vi "TLB Native Dynamic Events ver 0.10.vi"() -> ()   [LabVIEW 2018]
uses:
  Labview Training Phase 2/Enum Controls/States for Action Engine.ctl
  TLB Type Definitions/State Type Definitions.ctl
  TLB Type Definitions/Intruction Type Definitions.ctl
  TLB Type Definitions/Encoder cluster.ctl
  Experimental VI's/Archived VI's/MOTOR CONTROL NO PID Type Def.ctl
  Underlying VI's/I2C Master VI/I2C MASTER Type Def.ctl
  TLB Type Definitions/PING CLUSTER.ctl
  <vilib>/Studica/Studica Toolkit/NavX/NavX.lvlib
  <vilib>/Studica/Studica Toolkit/Background/DIO Channel.ctl
panel:
  out "Object detected?":bool
  out "TASK ENABLE":bool
  out "Rising Edge":bool
  in  "Green LED":bool
  out "Timestamp":u32
  out "NavX Output":T1
  in  "Zero Yaw":bool
  out "Task Selection":u8
  out "Object detected?":bool
  in  "Arduino Mode":T2=enum."Mode 0"
  out "Arduino Data":T3
  out "I2C Error":errorcluster
  out "Speed & distance":T4
  out "State Logic":T5=enum."Startup"
  out "elements":T6[](array[typedef])
  in  "STOP TASK":bool
  in  "OK Button":bool
  in  "STOP":bool
  out "error out":errorcluster
  out "Action Queue Items":i32
  out "State Logic Queue Items":i32
  out "Action Queues items":string[](array[string])=["Hardware reset", "Software reset", ""]
  out "Action State":string
  # "TLB FRAMEWORK STATUS"
  # "System Health Status Update"
  # "Test Programme written by Calvin Loke    Dated: 28 Aug 2019\nTest Programme revised by Dr Alex See   Dated 30 Aug 2019\n\nProgramme version:   TLB Native Dynamic Events ver 0.04b.vi"
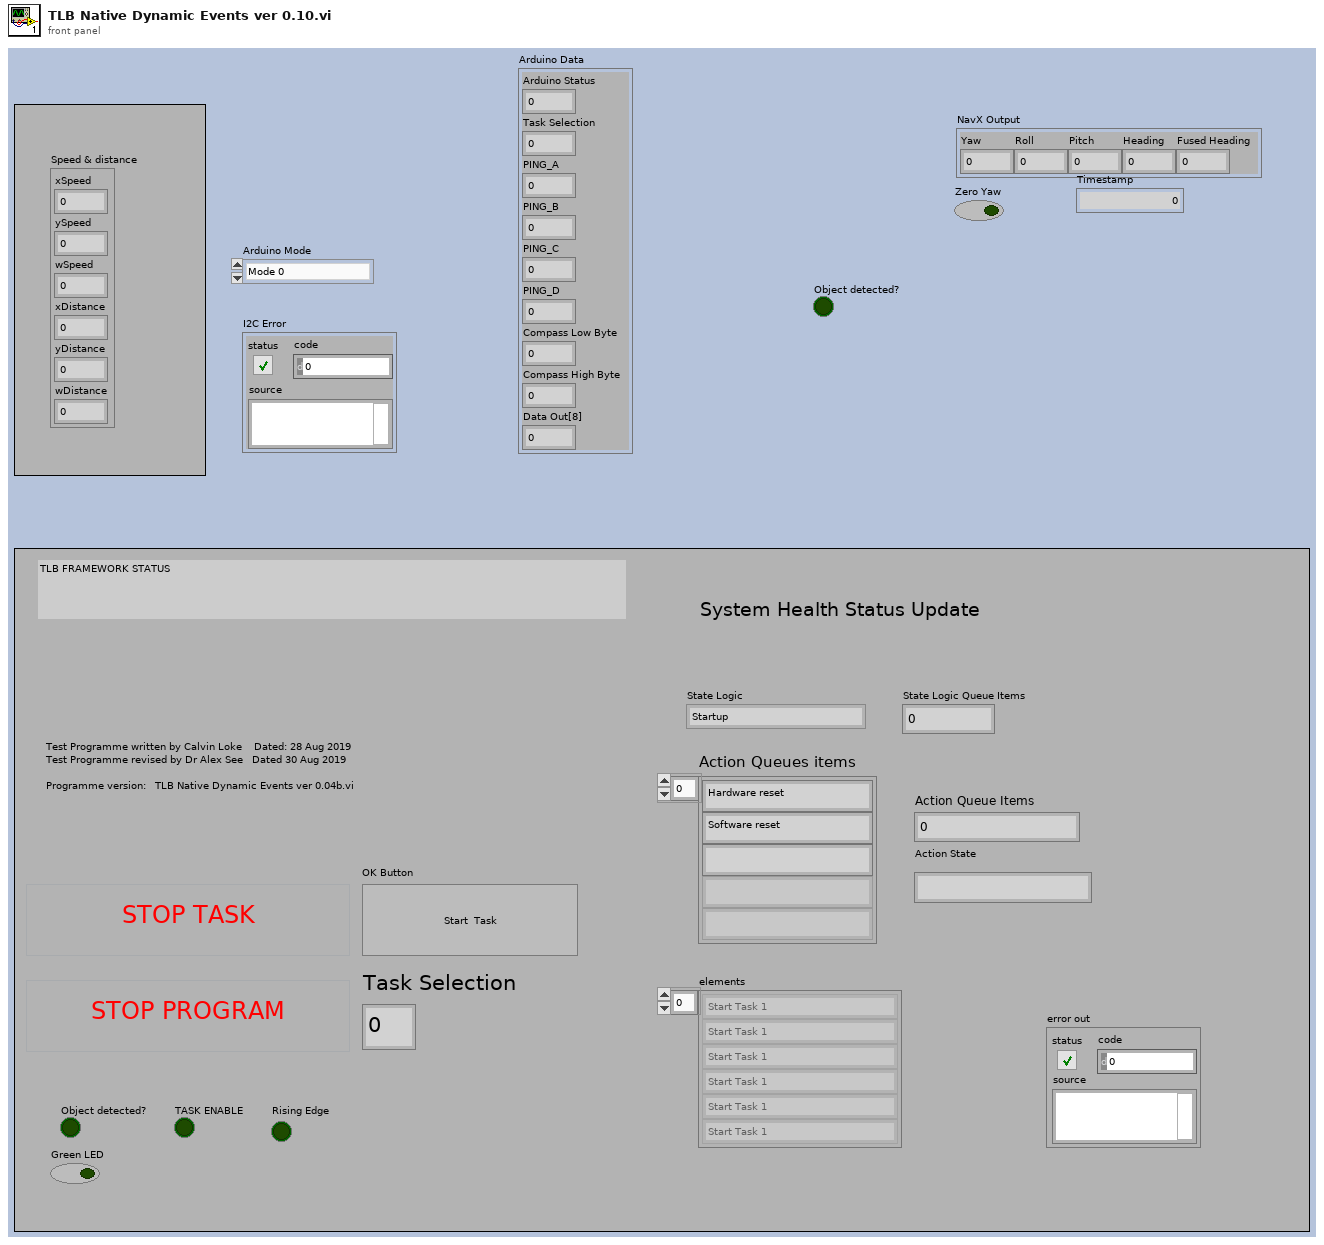
[diagram p1: front panel]
types:
  T1 = cluster{"Yaw":dbl, "Roll":dbl, "Pitch":dbl, "Heading":dbl, "Fused Heading":dbl}
  T2 = typedef "I2C MASTER Type Def.ctl" = enum16{"Last State", "Mode 0", "Mode 1", "Mode 2", "Mode 3", "Mode 4", "Mode 5", "Mode 6", "Mode 7", "Mode 8", "Mode 9", "Mode 10"}
  T3 = cluster{"Arduino Status":u8, "Task Selection":u8, "PING_A":u8, "PING_B":u8, "PING_C":u8, "PING_D":u8, "Compass Low Byte":u8, "Compass High Byte":u8, "Data Out[8]":u8}
  T4 = cluster{"xSpeed":dbl, "ySpeed":dbl, "wSpeed":dbl, "xDistance":dbl, "yDistance":dbl, "wDistance":dbl}
  T5 = typedef "State Type Definitions.ctl" = enum16{"None", "Startup", "Move to Angle", "True Stop", "Idle", "Shutdown", "Task 1A", "Task 1B", "Task 2:Raise Arm", "Task 2:Sensor Mode", "Task 2:Reverse Mode", "Task 3", "Task 4_A", "Task 4_B", "Task 4_C", "Task 4_D", "Task 5A", "Task 5B", "Task 5C", "Task 5D", "Task 5E: POSITION ARM", "Task 5F: ARM GRAB HEIGHT", "Task 5G: CLOSE CLAW", "Task 5H: RAISE ARM", "Task 6_A", "Task 6_B", "Task 7", "Task 8A: RAISE ARM", "Task 8B: MOVE TO BOX", "Task 8C: CAM BURST", "Task 8D: PROCESS IMAGE", "Task 8E: ROBOT ADJUST", "Task 8F: CAM BURST 2", "Task 8G: PROCESS IMAGE 2", "Task 8H: ARM ADJUST", "Task 8I: ARM GRAB HEIGHT", "Task 8J: CLOSE CLAW", "Task 8K: RAISE MY SWORD", "Task 9A: Raise Arm", "Task 9B: Rotate to Angle", "Task 9C: Detect Box", "Task 9D: MOVE FORWARD", "Task 9E: MOVE LEFT", "Task 9F: SCAN IMAGE", "Task 9G: PROCESS COLOUR", "Task 9H: MOVE RIGHT", "Task 9I: SCAN IMAGE", "Task 9J: PROCESS COLOUR", "Task 9K: ROTATE 90 CW", "Task 9L: MOVE FORWARD", "Task 9M: MOVE RIGHT", "Task 9N: SCAN IMAGE", "Task 9O: PROCESS COLOUR", "Task 9P: MOVE RIGHT", "Task 9Q: SCAN IMAGE", "Task 9R: PROCESS COLOUR"}
  T6 = typedef "Intruction Type Definitions.ctl" = enum16{"None", "Start Task 1", "Start Task 2", "Start Task 3", "Start Task 4", "Start Task 5", "Start Task 6", "Start Task 7", "Start Task 8 - BALL", "Start Task 8 - Gel", "Start Task 8 - Pipe", "Start Task 8 - Soap", "Start Task 9", "Start Task A", "Start Task B", "Exit"}
  T7 = typedef "States for Action Engine.ctl" = enum16{"Initialize", "Write", "Read"}
  T8 = typedef "DIO Channel.ctl" = enum16{"Not Connected", "A/DIO1", "A/DIO2", "A/DIO3", "A/DIO4", "A/DIO5", "A/DIO6", "A/DIO7", "A/DIO13", "B/DIO1", "B/DIO2", "B/DIO3", "B/DIO4", "B/DIO5", "B/DIO6", "B/DIO7", "B/DIO13", "C/DIO0", "C/DIO1", "C/DIO2", "C/DIO3", "C/DIO4", "C/DIO5", "C/DIO6", "C/DIO7"}
  T9 = typedef "PING CLUSTER.ctl" = cluster{"PING_A":u8, "PING_B":u8, "PING_C":u8, "PING_D":u8}
  T10 = typedef "Encoder cluster.ctl" = cluster{"xDistance":dbl, "yDistance":dbl, "wDistance":dbl}
  T11 = typedef "State Type Definitions.ctl" = enum16{"None", "Startup", "Move to Angle", "True Stop", "Idle", "Shutdown", "Task 1", "Task 2:Raise Arm", "Task 2:Sensor Mode", "Task 2:Reverse Mode", "Task 3", "Task 4_A", "Task 4_B", "Task 4_C", "Task 4_D", "Task 5A: ARM CAM HEIGHT", "Task 5B: MOVE TO BOX", "Task 5C: CAM BURST", "Task 5D: PROCESS IMAGE", "Task 5E: POSITION ARM", "Task 5F: ARM GRAB HEIGHT", "Task 5G: CLOSE CLAW", "Task 5H: RAISE ARM", "Task 6_A", "Task 6_B", "Task 7", "Task 8A: RAISE ARM", "Task 8B: MOVE TO BOX", "Task 8C: CAM BURST", "Task 8D: PROCESS IMAGE", "Task 8E: ROBOT ADJUST", "Task 8F: CAM BURST 2", "Task 8G: PROCESS IMAGE 2", "Task 8H: ARM ADJUST", "Task 8I: ARM GRAB HEIGHT", "Task 8J: CLOSE CLAW", "Task 8K: RAISE MY SWORD", "Task 9A: Raise Arm", "Task 9B: Rotate to Angle", "Task 9C: Detect Box", "Task 9D: MOVE FORWARD", "Task 9E: MOVE LEFT", "Task 9F: SCAN IMAGE", "Task 9G: PROCESS COLOUR", "Task 9H: MOVE RIGHT", "Task 9I: SCAN IMAGE", "Task 9J: PROCESS COLOUR", "Task 9K: ROTATE 90 CW", "Task 9L: MOVE FORWARD", "Task 9M: MOVE RIGHT", "Task 9N: SCAN IMAGE", "Task 9O: PROCESS COLOUR", "Task 9P: MOVE RIGHT", "Task 9Q: SCAN IMAGE", "Task 9R: PROCESS COLOUR"}
  T12 = typedef "State Type Definitions.ctl" = enum16{"None", "Startup", "Move to Angle", "True Stop", "Idle", "Shutdown", "Task 1", "Task 2", "Task 3", "Task 4_A", "Task 4_B", "Task 4_C", "Task 5", "Task 6", "Task 7", "Task 8", "Task 9", "Task A", "Task B"}
  T13 = typedef "MOTOR CONTROL NO PID Type Def.ctl" = enum16{"Init", "Front Back", "Left Right", "Rotate", "Stop", "Latch"}
  T14 = cluster{"DIO Channel":T8, "FPGA VI Reference Out":refnum<k20>}
  T15 = typedef "I2C Channel.ctl" = enum16{"Not Connected", "A", "B"}
  T16 = cluster{"I2C Ref Out":cluster{"I2C Channel":T15, "FPGA VI Reference Out":refnum<k20>}, "Connected":bool, "Slave Address (7-bit)":u8, "Registry":u8[]}
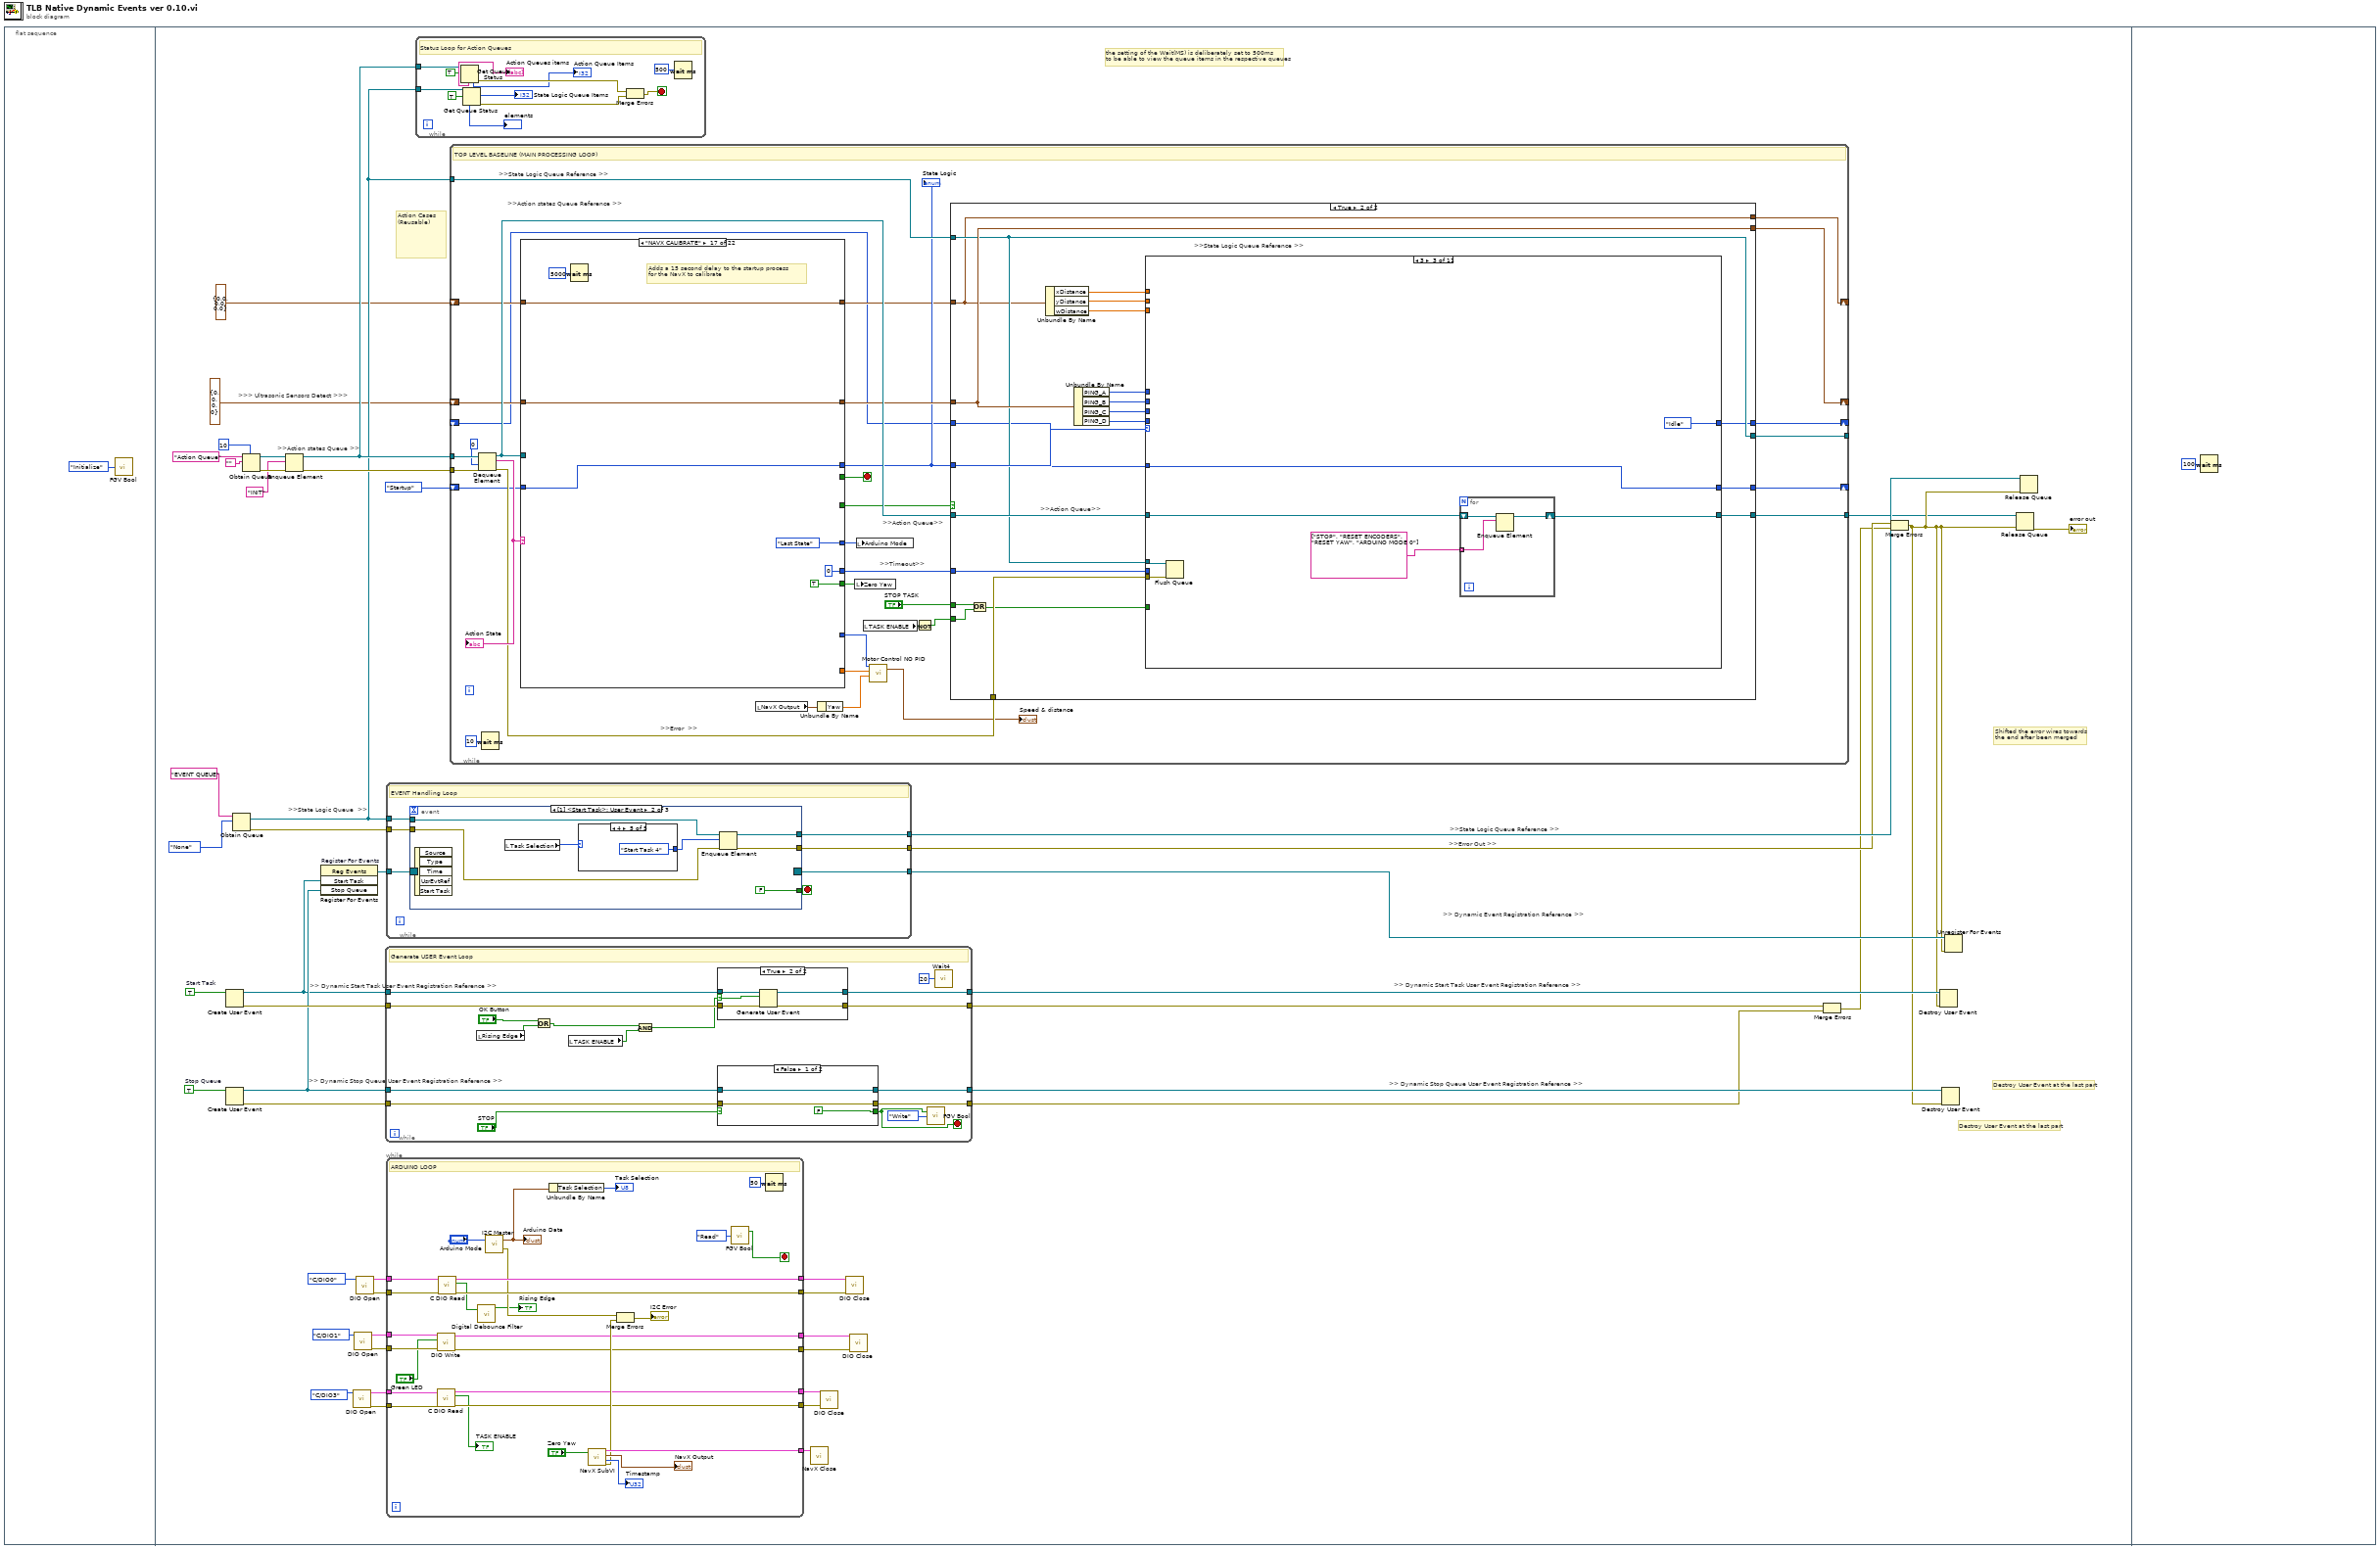
[diagram p0: block diagram]
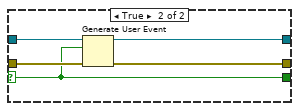
[diagram p2: hidden frame]
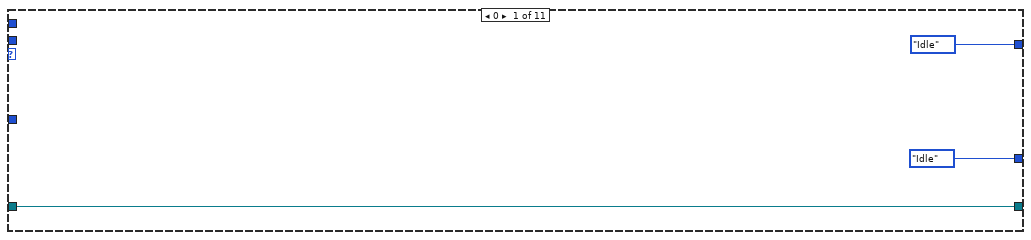
[diagram p5: hidden frame]
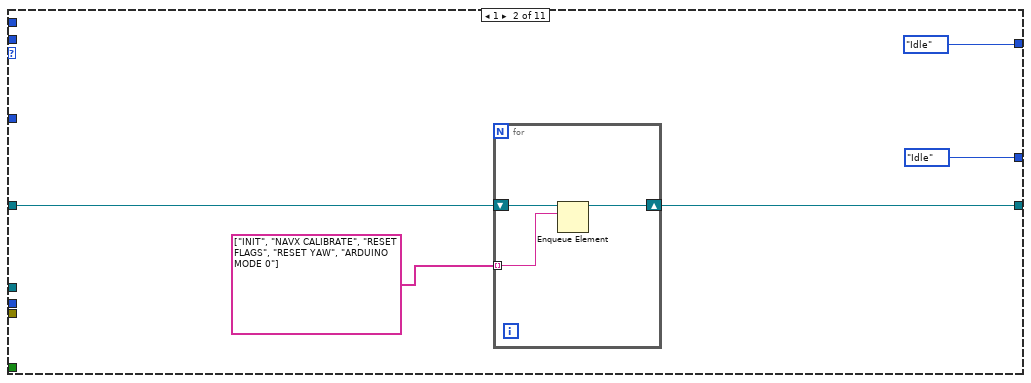
[diagram p6: hidden frame]
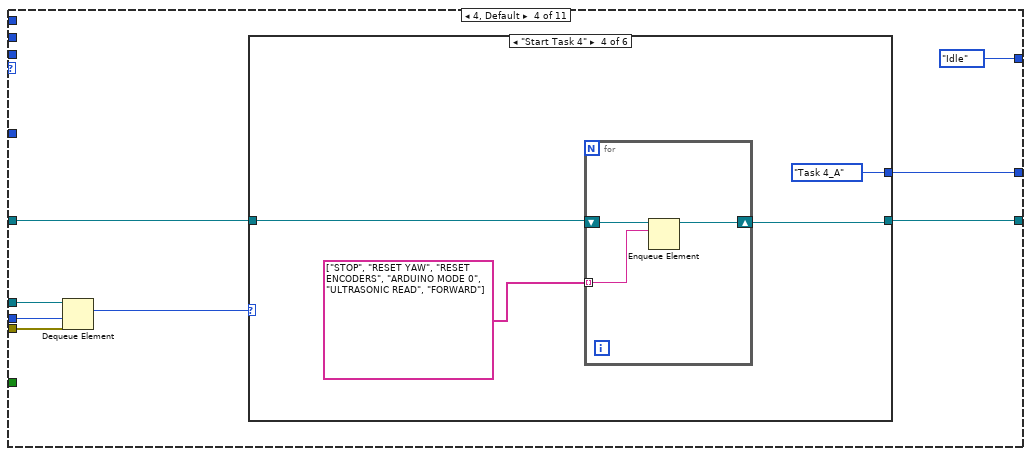
[diagram p7: hidden frame]
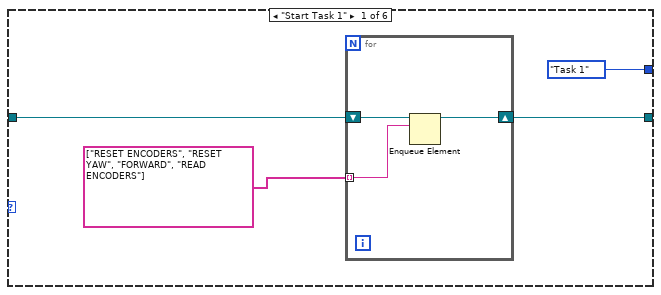
[diagram p8: hidden frame]
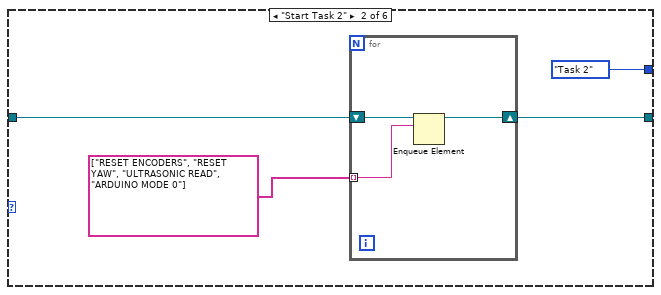
[diagram p9: hidden frame]
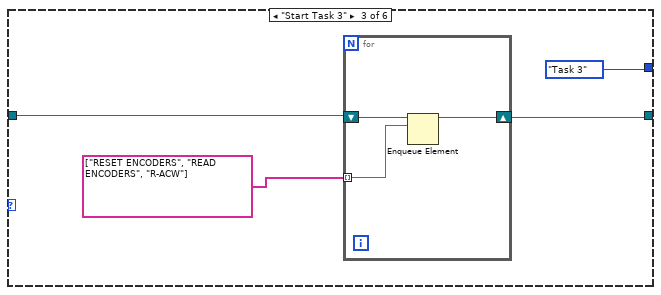
[diagram p10: hidden frame]
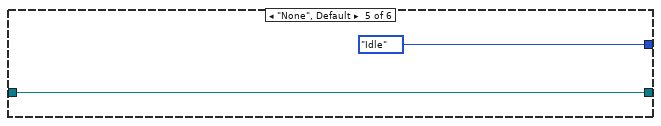
[diagram p11: hidden frame]
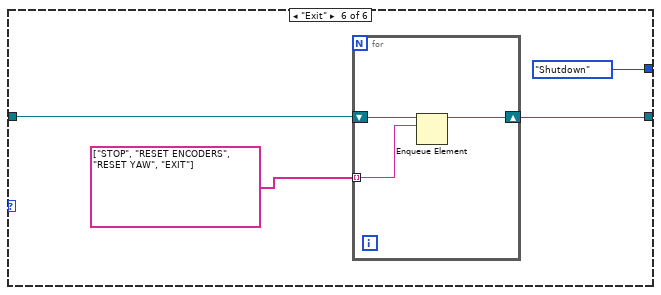
[diagram p12: hidden frame]
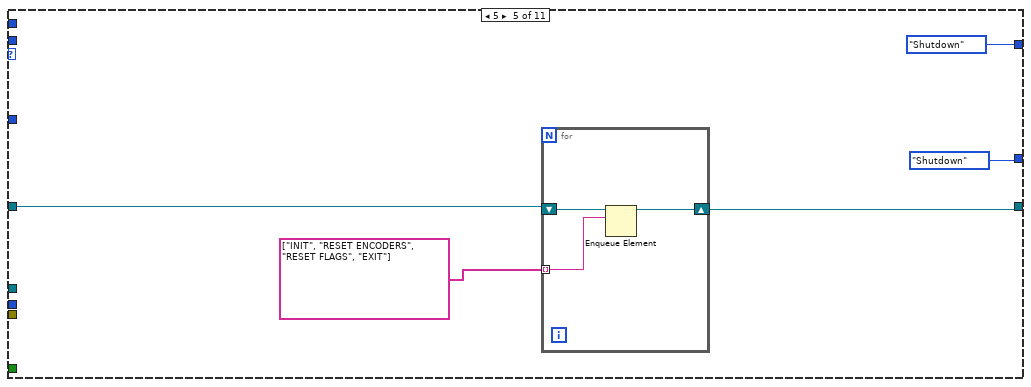
[diagram p13: hidden frame]
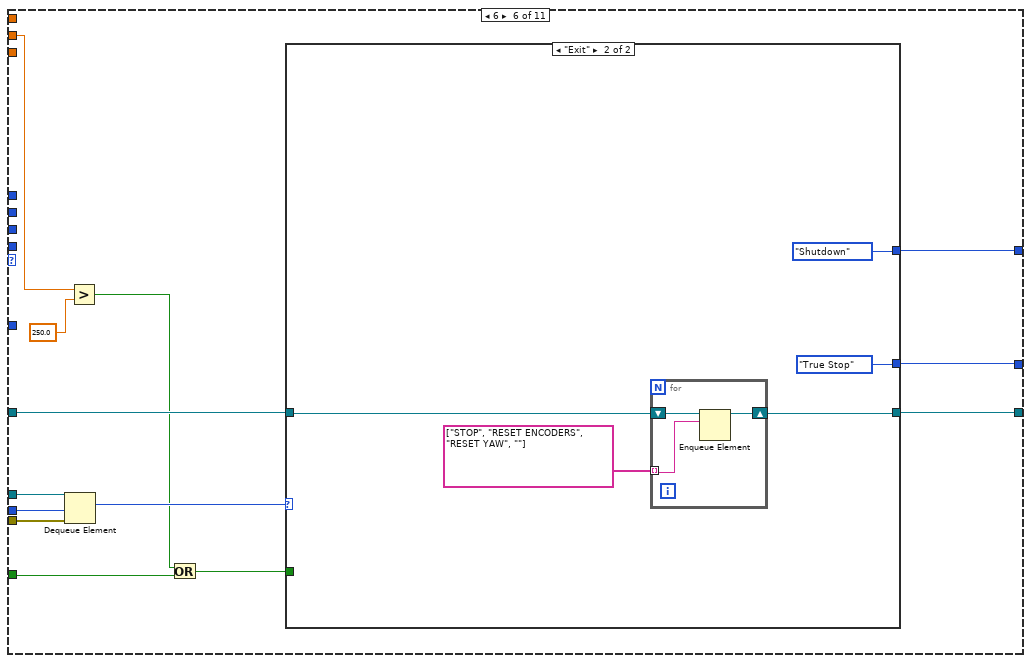
[diagram p14: hidden frame]
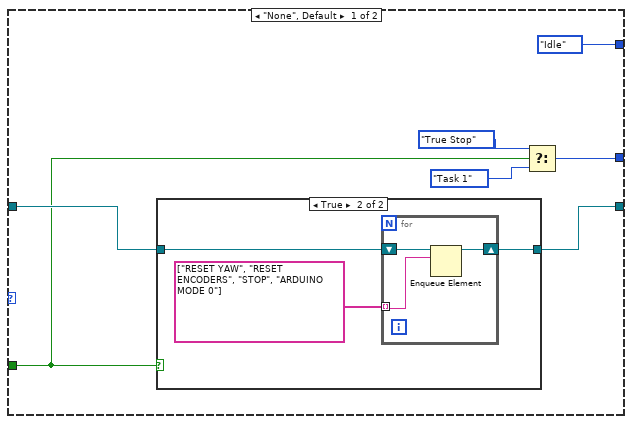
[diagram p15: hidden frame]
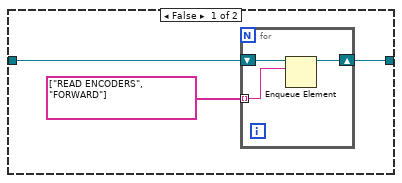
[diagram p16: hidden frame]
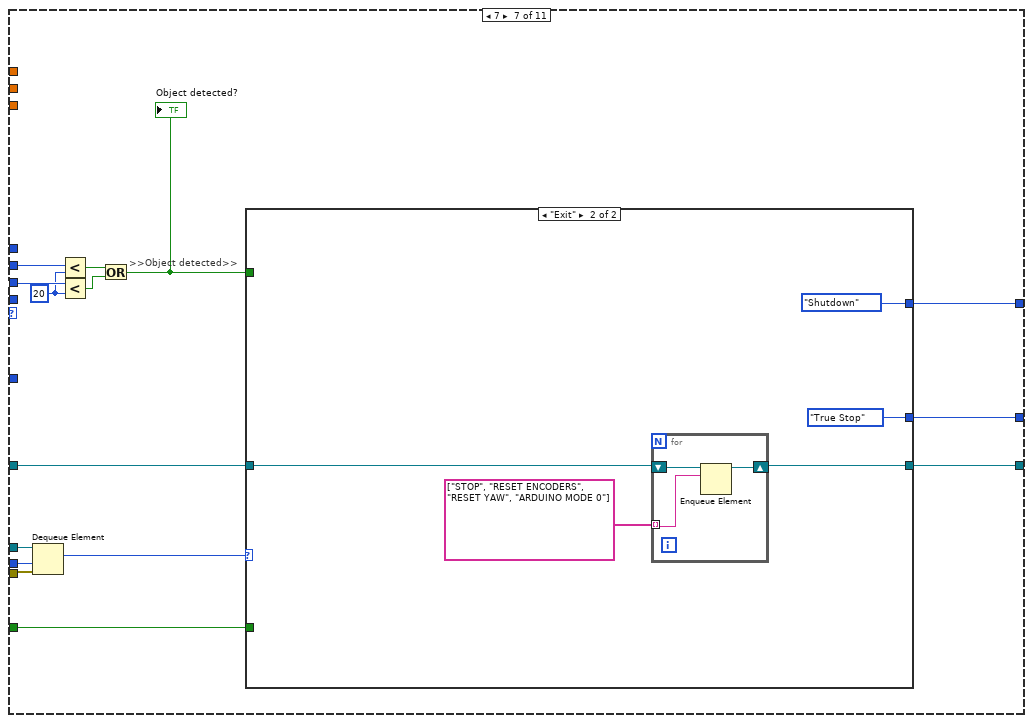
[diagram p17: hidden frame]
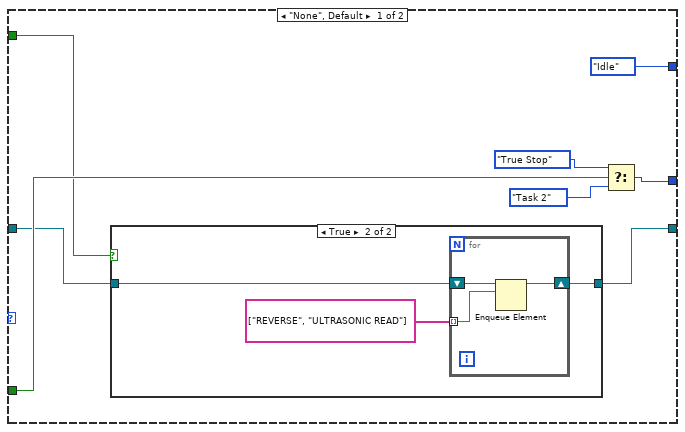
[diagram p18: hidden frame]
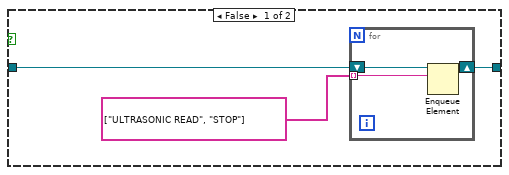
[diagram p19: hidden frame]
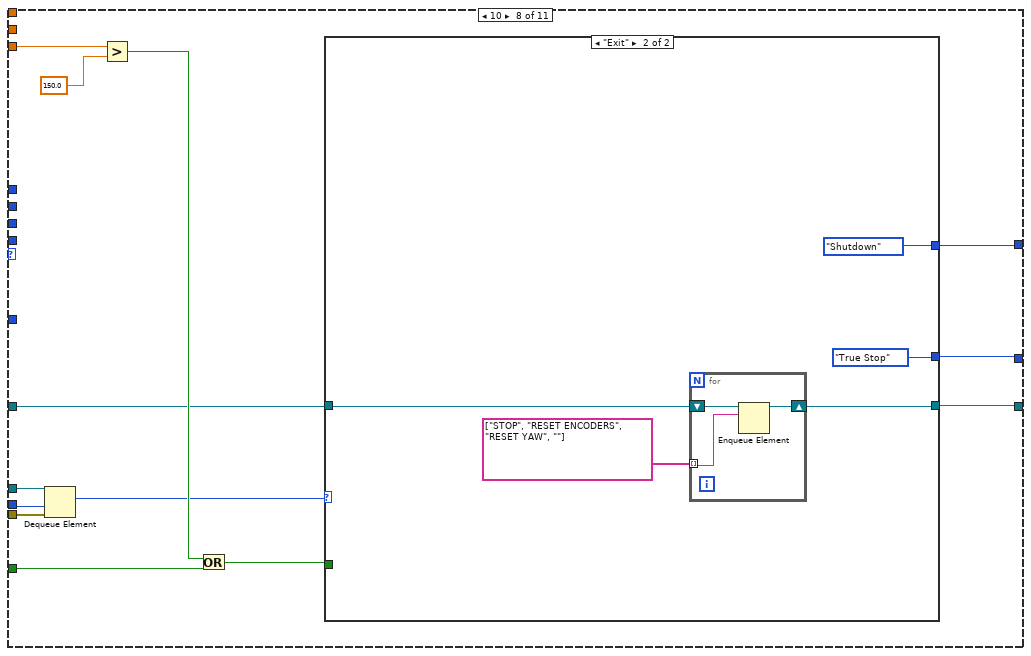
[diagram p20: hidden frame]
diagram:
  n1 = flat-sequence {
    frame #0 {
      n2 = call "FGV Bool.vi"("Init/Read/Write State"=States_for_Action_Engine."Initialize") -> ()  [unwired: 2 in, 2 out]
    }
    frame #1 {
      w50 = TRUE  # Stop Queue
      w49 = TRUE  # Start Task
      # ">>> Ultrasonic Sensors Detect >>>"
      # "the setting of the Wait(MS) is deliberately set to 500ms\nto be able to view the queue items in the respective queues"
      # "Action Cases\n(Reusable)"
      # ">>Error Out >>"
      # ">> Dynamic Stop Queue User Event Registration Reference >>"
      # ">> Dynamic Start Task User Event Registration Reference >>"
      # ">> Dynamic Stop Queue User Event Registration Reference >>"
      # ">> Dynamic Start Task User Event Registration Reference >>"
      # ">> Dynamic Event Registration Reference >>"
      # ">>Action states Queue >>"
      # ">>State Logic Queue  >>"
      # ">>State Logic Queue Reference >>"
      # "Destroy User Event at the last part"
      # "Destroy User Event at the last part"
      # "Shifted the error wires towards\nthe end after been merged"
      n3 = Create User Event(user event datatype=w49) -> (user event=w41:refnum<user-event>, error out=w46:errorcluster)  [unwired: 1 in]
      n4 = Create User Event(user event datatype=w50) -> (user event=w42:refnum<user-event>, error out=w45:errorcluster)  [unwired: 1 in]
      n5 = Obtain Queue(name (unnamed)="EVENT QUEUE", element data type=Intruction_Type_Definitions."None" ("Enum")) -> (queue out=w27:refnum<queue>, error out=w33:errorcluster)  [unwired: 3 in, 1 out]
      n6 = Obtain Queue(max queue size (-1, unlimited)=10, name (unnamed)="Action Queue", element data type="") -> (queue out=w36:refnum<queue>, error out=w32:errorcluster)  [unwired: 2 in, 1 out]
      n7 = Enqueue Element(queue=w36, element="INIT", error in (no error)=w32) -> (queue out=w28:refnum<queue>, error out=w31:errorcluster)  [unwired: 1 in, 1 out]
      n8 = register-events "Register For Events"(w41, w42) -> (reference out=w40:refnum<event-registration>)  [unwired: 2 in, 1 out]
      n9 = call <vilib>:"DIO Open.vi"("DIO Channel"=DIO_Channel."C/DIO3") -> ("error out"=w3:errorcluster, "DIO Info Out"=w4:T14)  [unwired: 9 in]
      n10 = call <vilib>:"DIO Open.vi"("DIO Channel"=DIO_Channel."C/DIO1") -> ("error out"=w8:errorcluster, "DIO Info Out"=w10:T14)  [unwired: 9 in]
      n11 = call <vilib>:"DIO Open.vi"("DIO Channel"=DIO_Channel."C/DIO0") -> ("error out"=w13:errorcluster, "DIO Info Out"=w16:T14)  [unwired: 9 in]
      n12 = while {
        tunnel: w41 -> [w108]
        tunnel: w42 -> [w107]
        tunnel: [w106] -> w48
        tunnel: [w105] -> w47
        tunnel: w46 -> [w104]
        tunnel: [w103] -> w44
        tunnel: w45 -> [w102]
        tunnel: [w101] -> w43
        stop <- w99 stop-if-true
        # "Generate USER Event Loop"
        n13 = local read "Rising Edge"() -> (w95:bool)
        n14 = Or(x="OK Button", y=w95) -> (x .or. y?=w94:bool)
        n15 = local read "TASK ENABLE"() -> (w93:bool)
        n16 = And(x=w94, y=w93) -> (x .and. y?=w92:bool)
        n17 = case shown="True" w92 {
          selector: w92 -> [_ w119]
          tunnel: w108 -> [w118 w123]
          tunnel: [w118 w122] -> w105
          tunnel: w104 -> [w117 w121]
          tunnel: [w117 w120] -> w103
          frame False {
          }
          frame True {
            n18 = Generate User Event(user event=w123, event data cluster=w119, error in=w121) -> (user event out=w122:refnum<user-event>, error out=w120:errorcluster)  [unwired: 1 in]
          }
        }
        n19 = case shown="False" "STOP" {
          selector: "STOP" -> [_ w112]
          tunnel: w107 -> [w111 w116]
          tunnel: [w111 w115] -> w106
          tunnel: w102 -> [w110 w114]
          tunnel: [w110 w113] -> w101
          tunnel: [FALSE w112] -> w99
          frame False {
          }
          frame True {
            n20 = Generate User Event(user event=w116, event data cluster=w112, error in=w114) -> (user event out=w115:refnum<user-event>, error out=w113:errorcluster)  [unwired: 1 in]
          }
        }
        n21 = call "FGV Bool.vi"("Init/Read/Write State"=States_for_Action_Engine."Write", "Input Node"=w99) -> ()  [unwired: 1 in, 2 out]
        n22 = call "Wait4"("Count(uSec)"=u32 20) -> ()  [unwired: 1 out]
      }
      n23 = while {
        tunnel: w40 -> [w668]
        tunnel: [w667] -> w39
        tunnel: w27 -> [w665]
        tunnel: [w664] -> w38
        tunnel: w33 -> [w663]
        tunnel: [w662] -> w30
        stop <- w666 stop-if-true
        # "EVENT Handling Loop"
        n24 = event shown="[1] <Start Task>: User Event" {
          selector: w668 -> [_ _ _]
          dyn-events: [_ _ _] -> w667
          timeout: _ -> [_ _ _]
          tunnel: [FALSE FALSE w692] -> w666
          tunnel: w665 -> [w673 w680 w690]
          tunnel: [w672 w679 w691] -> w664
          tunnel: w663 -> [w671 w678 w689]
          tunnel: [w670 w677 w688] -> w662
          event Timeout {
            n25 = event-data() -> ()  [unwired: 1 in, 3 out]
            n26 = Enqueue Element(queue=w673, element=Intruction_Type_Definitions."None" ("Enum"), error in (no error)=w671) -> (queue out=w672:refnum<queue>, error out=w670:errorcluster)  [unwired: 1 in, 1 out]
          }
          event User Event {
            n27 = event-data() -> ()  [unwired: 1 in, 5 out]
            n28 = local read "Task Selection"() -> (w675:u8)
            n29 = case shown="4" w675 {
              tunnel: [Intruction_Type_Definitions."None" ("Enum") Intruction_Type_Definitions."Start Task 1" ("Enum") Intruction_Type_Definitions."Start Task 2" ("Enum") Intruction_Type_Definitions."Start Task 3" ("Enum") Intruction_Type_Definitions."Start Task 4" ("Enum")] -> w676
              frame 0, Default {
              }
              frame 1 {
              }
              frame 2 {
              }
              frame 3 {
              }
              frame 4 {
              }
            }
            n30 = Enqueue Element(queue=w680, element=w676, error in (no error)=w678) -> (queue out=w679:refnum<queue>, error out=w677:errorcluster)  [unwired: 1 in, 1 out]
          }
          event User Event {
            n31 = event-data() -> ("Stop Queue"=w692:bool)  [unwired: 1 in, 4 out]
            n32 = Enqueue Element At Opposite End(queue=w690, element=Intruction_Type_Definitions."Exit" ("Enum"), error in (no error)=w689) -> (queue out=w691:refnum<queue>, error out=w688:errorcluster)  [unwired: 1 in, 1 out]
          }
        }
      }
      n33 = while {
        tunnel: [w71] -> w17
        tunnel: w16 -> [w70]
        tunnel: [w69] -> w14
        tunnel: w13 -> [w68]
        tunnel: [w67] -> w12
        tunnel: w10 -> [w60]
        tunnel: [w59] -> w9
        tunnel: w8 -> [w58]
        tunnel: [w57] -> w7
        tunnel: [w55] -> w5
        tunnel: w4 -> [w54]
        tunnel: w3 -> [w53]
        tunnel: [w52] -> w2
        stop <- w78 stop-if-true
        # "ARDUINO LOOP"
        n34 = call <vilib>:"DIO Write.vi"("error in (no error)"=w58, "Input"="Green LED", "DIO Info In"=w60) -> ("error out"=w57:errorcluster, "DIO Info Out"=w59:T14)  [unwired: 7 in]
        n35 = call <vilib>:"C DIO Read.vi"("error in (no error)"=w53, "DIO Info In in"=w54) -> ("error out"=w52:errorcluster, "IN"=→"TASK ENABLE":bool, "DIO Info In out"=w55:T14)  [unwired: 7 in]
        n36 = call <vilib>:"C DIO Read.vi"("error in (no error)"=w68, "DIO Info In in"=w70) -> ("error out"=w67:errorcluster, "IN"=w63:bool, "DIO Info In out"=w69:T14)  [unwired: 7 in]
        n37 = call "Digital Debounce Filter.vi"("Boolean input"=w63) -> ("Rising Edge"=→"Rising Edge":bool)  [unwired: 1 in, 2 out]
        n38 = call "I2C Master.vi"("Arduino Mode"="Arduino Mode") -> ("I2C Error"=w66:errorcluster, "Arduino Data"=w61:T3)  [unwired: 1 in]
        "Arduino Data" <- w61
        n39 = Unbundle By Name(w61) -> ("Task Selection"=→"Task Selection":u8)
        n40 = call "NavX SubVI.vi"("Zero Yaw"="Zero Yaw") -> ("NavX Info Out"=w71:T16, "NavX Output"=→"NavX Output":T1, "Timestamp"=→"Timestamp":u32, "error out"=w65:errorcluster)  [unwired: 1 in]
        n41 = Merge Errors(w66, w65) -> (→"I2C Error":errorcluster)
        n42 = call "FGV Bool.vi"("Init/Read/Write State"=States_for_Action_Engine."Read") -> ("Output node"=w78:bool)  [unwired: 2 in, 1 out]
        n43 = Wait (ms)(milliseconds to wait=u32 50) -> ()  [unwired: 1 out]
      }
      n44 = while {
        tunnel: w28 -> [w89]
        tunnel: w27 -> [w86]
        stop <- w83 stop-if-true
        # "Status Loop for Action Queues"
        n45 = Get Queue Status(queue=w89, return elements? (F)=TRUE) -> (error out=w85:errorcluster, # elements in queue=→"Action Queue Items":i32, elements=→"Action Queues items":string[])  [unwired: 1 in, 5 out]
        n46 = Get Queue Status(queue=w86, return elements? (F)=TRUE) -> (# pending remove=→"State Logic Queue Items":i32, error out=w84:errorcluster, elements=→"elements":T6[])  [unwired: 1 in, 5 out]
        n47 = Merge Errors(w85, w84) -> (w83:errorcluster)
        n48 = Wait (ms)(milliseconds to wait=u32 500) -> ()  [unwired: 1 out]
      }
      n49 = while {
        tunnel: w27 -> [w145]
        tunnel: w28 -> [w157]
        tunnel: w31 -> [w155]
        tunnel: [w154] -> _
        tunnel: [w153] -> w20
        shift-right: [w146] -> _
        shift-left: T9 {"PING_A"=0, "PING_B"=0, "PING_C"=0, "PING_D"=0} -> [w148]
        shift-right: [w139] -> _
        shift-left: State_Type_Definitions."Startup" ("Enum") -> [w142]
        shift-right: [w135] -> _
        shift-left: T10 {"xDistance"=0.0, "yDistance"=0.0, "wDistance"=0.0} -> [w137]
        shift-right: [w126] -> _
        shift-left: _ -> [w125]
        stop <- w144 stop-if-true
        # ">>Error  >>"
        # ">>Action Queue>>"
        # ">>Timeout>>"
        # ">>Action states Queue Reference >>"
        # ">>State Logic Queue Reference >>"
        # "TOP LEVEL BASELINE (MAIN PROCESSING LOOP)"
        n50 = Dequeue Element(queue=w157, timeout in ms (-1)=0, error in (no error)=w155) -> (queue out=w149:refnum<queue>, element=w156:string, error out=w150:errorcluster)  [unwired: 1 out]
        "Action State" <- w156
        n51 = Wait (ms)(milliseconds to wait=u32 10) -> ()  [unwired: 1 out]
        n52 = case shown="\"NAVX CALIBRATE\"" w156 {
          tunnel: [_ _ _ _ _ _ _ _ _ _ _ _ _ _ _ _ 0 w635 _ _ _ _] -> w152
          tunnel: w149 -> [_ _ _ _ _ _ _ _ _ _ _ _ _ _ _ _ _ _ _ _ _ _]
          tunnel: w148 -> [w532 w537 w543 w548 w554 w559 w564 w570 w576 w579 w590 w600 w604 w613 w617 w621 w629 w636 w641 w646 w653 w661]
          tunnel: [w532 w537 w543 w548 w554 w559 w564 w570 w576 w579 w590 w601 w604 w614 w617 w621 w629 w636 w641 w646 w652 w661] -> w147
          tunnel: [TRUE TRUE _ _ _ _ _ _ _ _ _ _ _ _ _ _ _ _ _ _ _ _] -> w144
          tunnel: w142 -> [w530 w535 w542 w547 w553 w558 w563 w569 w575 w578 w589 w599 w603 w612 w616 w620 w626 w633 w640 w645 w651 w660]
          tunnel: [_ _ _ _ _ _ _ _ _ _ _ _ _ _ _ _ _ TRUE _ _ _ _] -> w141
          tunnel: [w530 w535 w542 w547 w553 w558 w563 w569 w575 w578 w589 w599 w603 w612 w616 w620 w626 w633 w640 w645 w651 w660] -> w140
          tunnel: w137 -> [w529 w534 w541 w546 w552 w557 w562 w568 w574 w580 w588 w598 w605 w611 w618 w622 w625 w632 w642 w647 w650 w659]
          tunnel: [w529 w534 w541 w546 w552 w557 w562 w568 w574 w580 w587 w598 w605 w610 w618 w622 w625 w632 w642 w647 w650 w659] -> w136
          tunnel: [_ _ 0.4 ("Speed") -0.3 ("Speed") 0.19999999999999998 ("Speed") -0.2 ("Speed") _ 0.3 ("Speed") -0.5 ("Speed") _ _ _ _ 0.0 ("Speed") _ _ _ _ _ _ _ _] -> w134
          tunnel: [_ _ MOTOR_CONTROL_NO_PID_Type_Def."Front Back" ("Direction") _ MOTOR_CONTROL_NO_PID_Type_Def."Rotate" ("Direction") _ MOTOR_CONTROL_NO_PID_Type_Def."Stop" ("Direction") MOTOR_CONTROL_NO_PID_Type_Def."Left Right" ("Direction") MOTOR_CONTROL_NO_PID_Type_Def."Front Back" ("Direction") _ MOTOR_CONTROL_NO_PID_Type_Def."Latch" ("Direction") MOTOR_CONTROL_NO_PID_Type_Def."Latch" ("Direction") _ _ _ _ _ MOTOR_CONTROL_NO_PID_Type_Def."Latch" ("Direction") _ MOTOR_CONTROL_NO_PID_Type_Def."Init" ("Direction") _ MOTOR_CONTROL_NO_PID_Type_Def."Init" ("Direction")] -> w132
          tunnel: [I2C_MASTER_Type_Def."Last State" ("Arduino Mode") I2C_MASTER_Type_Def."Last State" ("Arduino Mode") I2C_MASTER_Type_Def."Last State" ("Arduino Mode") I2C_MASTER_Type_Def."Last State" ("Arduino Mode") I2C_MASTER_Type_Def."Last State" ("Arduino Mode") I2C_MASTER_Type_Def."Last State" ("Arduino Mode") I2C_MASTER_Type_Def."Last State" ("Arduino Mode") I2C_MASTER_Type_Def."Last State" ("Arduino Mode") I2C_MASTER_Type_Def."Last State" ("Arduino Mode") I2C_MASTER_Type_Def."Last State" ("Arduino Mode") I2C_MASTER_Type_Def."Last State" ("Arduino Mode") I2C_MASTER_Type_Def."Mode 0" ("Arduino Mode") I2C_MASTER_Type_Def."Last State" ("Arduino Mode") I2C_MASTER_Type_Def."Last State" ("Arduino Mode") I2C_MASTER_Type_Def."Mode 0" ("Arduino Mode") I2C_MASTER_Type_Def."Mode 1" ("Arduino Mode") I2C_MASTER_Type_Def."Last State" ("Arduino Mode") I2C_MASTER_Type_Def."Last State" ("Arduino Mode") I2C_MASTER_Type_Def."Last State" ("Arduino Mode") I2C_MASTER_Type_Def."Last State" ("Arduino Mode") I2C_MASTER_Type_Def."Last State" ("Arduino Mode") I2C_MASTER_Type_Def."Last State" ("Arduino Mode")] -> w131
          tunnel: [_ _ _ _ _ _ _ _ _ _ _ _ _ _ _ _ TRUE ("Zero Yaw") _ _ _ _ TRUE ("Zero Yaw")] -> w129
          frame "Exit" {
          }
          frame "----Movement States----" {
          }
          frame "FORWARD" {
          }
          frame "LEFT" {
          }
          frame "R-ACW" {
          }
          frame "R-CW" {
          }
          frame "STOP" {
          }
          frame "RIGHT" {
          }
          frame "REVERSE" {
          }
          frame "----SENSOR READING---- " {
          }
          frame "READ ENCODERS" {
            # ">>> Current encoder distance >>>"
            # ">>> Ultrasonic Sensors Detect >>>"
            n53 = local read "Speed & distance"() -> (w586:T4)
            n54 = Unbundle By Name(w586) -> ("xDistance"=w585:dbl, "yDistance"=w584:dbl, "wDistance"=w583:dbl)
            n55 = Bundle By Name(cluster=w588, "xDistance"=w585, "yDistance"=w584, "wDistance"=w583) -> (w587:T10)
          }
          frame "ULTRASONIC READ" {
            # "Object detection"
            n56 = local read "Arduino Data"() -> (w596:T3)
            n57 = Unbundle By Name(w596) -> ("PING_A"=w595:u8, "PING_B"=w594:u8, "PING_C"=w593:u8, "PING_D"=w592:u8)
            n58 = Bundle By Name(cluster=w600, "PING_A"=w595, "PING_B"=w594, "PING_C"=w593, "PING_D"=w592) -> (w601:T9)
          }
          frame "----SYSTEM MODES----" {
          }
          frame "INIT" {
            w607 = 0
            w609 = 0.0
            # ">>State Logic  >>"
            n59 = Bundle By Name(cluster=w613, "PING_A"=w607, "PING_B"=w607, "PING_C"=w607, "PING_D"=w607) -> (w614:T9)
            n60 = Bundle By Name(cluster=w611, "xDistance"=w609, "yDistance"=w609, "wDistance"=w609) -> (w610:T10)
          }
          frame "ARDUINO MODE 0" {
          }
          frame "ARDUINO MODE 1" {
          }
          frame "NAVX CALIBRATE" {
            # "Adds a 15 second delay to the startup process \nfor the NavX to calibrate"
            n61 = Wait (ms)(milliseconds to wait=u32 5000) -> ()  [unwired: 1 out]
          }
          frame "NO ACTION", Default {
            n62 = case shown="4" w633 {
              tunnel: [0 100] -> w635
              frame 1, Default {
              }
              frame 4 {
              }
            }
          }
          frame "----RESET CASES----" {
          }
          frame "RESET ENCODERS" {
          }
          frame "RESET FLAGS" {
            w649 = 0
            # "Resets any software variables\nand/or non-critical states"
            n63 = Wait (ms)(milliseconds to wait=u32 20) -> ()  [unwired: 1 out]
            n64 = Bundle By Name(cluster=w653, "PING_A"=w649, "PING_B"=w649, "PING_C"=w649, "PING_D"=w649) -> (w652:T9)
          }
          frame "RESET YAW" {
            n65 = Wait (ms)(milliseconds to wait=u32 1000) -> ()  [unwired: 1 out]
          }
        }
        "State Logic" <- w140
        n66 = local read "NavX Output"() -> (w130:T1)
        n67 = Unbundle By Name(w130) -> ("Yaw"=w124:dbl)
        n68 = local write "Zero Yaw"(w129) -> ()
        n69 = local write "Arduino Mode"(w131) -> ()
        n70 = local read "TASK ENABLE"() -> (w128:bool)
        n71 = call "Motor Control NO PID.vi"("Yaw"=w124, "Speed"=w134, "Direction"=w132) -> ("Speed & distance"=→"Speed & distance":T4)  [unwired: 1 in, 1 out]
        n72 = Not(x=w128) -> (.not. x?=w127:bool)
        n73 = case shown="True" w141 {
          tunnel: w145 -> [w163 w179]
          tunnel: w149 -> [w159 w181]
          tunnel: [w163 w179] -> w154
          tunnel: [w159 w182] -> w153
          tunnel: w150 -> [_ w177]
          tunnel: w152 -> [_ w178]
          tunnel: w147 -> [w162 w184]
          tunnel: [w162 w184] -> w146
          tunnel: "STOP TASK" -> [_ w167]
          tunnel: w140 -> [w161 w183]
          tunnel: [w161 w180] -> w139
          tunnel: w136 -> [w160 w173]
          tunnel: [w160 w173] -> w135
          tunnel: w127 -> [_ w168]
          tunnel: [w158 w165] -> w126
          tunnel: w125 -> [w158 w164]
          frame False {
          }
          frame True {
            # ">>Action Queue>>"
            # ">>State Logic Queue Reference >>"
            n74 = Or(x=w167, y=w168) -> (x .or. y?=w166:bool)
            n75 = Unbundle By Name(w173) -> ("xDistance"=w170:dbl, "yDistance"=w171:dbl, "wDistance"=w172:dbl)
            n76 = Unbundle By Name(w184) -> ("PING_A"=w176:u8, "PING_B"=w175:u8, "PING_C"=w174:u8, "PING_D"=w169:u8)
            n77 = case shown="3" w183 {
              tunnel: [w186 w189 w200 w207 w252 w264 w300 w346 w390 w447 w484] -> w182
              tunnel: w181 -> [w186 w192 w201 w210 w254 w265 w301 w347 w396 w440 w481]
              tunnel: [State_Type_Definitions."Idle" ("Enum") State_Type_Definitions."Idle" ("Enum") w196 w209 State_Type_Definitions."Shutdown" ("Enum") w266 w303 w345 w391 w446 w483] -> w180
              tunnel: w179 -> [_ _ w199 w213 _ w271 w313 w354 w395 w444 w482]
              tunnel: w178 -> [_ _ _ w212 _ w270 w312 w353 w394 w443 _]
              tunnel: w177 -> [_ _ w198 w208 _ w269 w311 w352 w393 w442 _]
              tunnel: w166 -> [_ _ _ _ _ w263 w302 w349 w389 w445 w486]
              tunnel: w176 -> [_ _ _ _ _ _ _ _ _ _ _]
              tunnel: w175 -> [_ _ _ _ _ _ w309 _ w387 w435 w488]
              tunnel: w174 -> [_ _ _ _ _ _ w308 _ w388 w436 w487]
              tunnel: w172 -> [_ _ _ _ _ _ _ w351 _ _ _]
              tunnel: w171 -> [_ _ _ _ _ w262 _ _ _ _ _]
              tunnel: w170 -> [_ _ _ _ _ _ _ _ _ w431 _]
              tunnel: w169 -> [_ _ _ _ _ _ _ _ _ _ _]
              tunnel: [State_Type_Definitions."Idle" ("Enum") State_Type_Definitions."Idle" ("Enum") State_Type_Definitions."Idle" ("Enum") State_Type_Definitions."Idle" ("Enum") State_Type_Definitions."Shutdown" ("Enum") w259 w299 w342 w382 w430 w485] -> w165
              tunnel: w164 -> [_ _ w196 _ _ _ _ _ _ _ _]
              frame 0 {
              }
              frame 1 {
                n78 = for {
                  shift-right: [w195] -> w189
                  shift-left: w192 -> [w194]
                  tunnel: string[] ["INIT", "NAVX CALIBRATE", "RESET FLAGS", "RESET YAW", "ARDUINO MODE 0"] -> [w193] mode=indexing
                  n79 = Enqueue Element(queue=w194, element=w193) -> (queue out=w195:refnum<queue>)  [unwired: 2 in, 2 out]
                }
              }
              frame 3 {
                n80 = Flush Queue(queue=w199, error in (no error)=w198) -> ()  [unwired: 3 out]
                n81 = for {
                  shift-right: [w205] -> w200
                  shift-left: w201 -> [w204]
                  tunnel: string[] ["STOP", "RESET ENCODERS", "RESET YAW", "ARDUINO MODE 0"] -> [w203] mode=indexing
                  n82 = Enqueue Element(queue=w204, element=w203) -> (queue out=w205:refnum<queue>)  [unwired: 2 in, 2 out]
                }
              }
              frame 4, Default {
                n83 = Dequeue Element(queue=w213, timeout in ms (-1)=w212, error in (no error)=w208) -> (element=w211:T6)  [unwired: 3 out]
                n84 = case shown="\"Start Task 4\"" w211 {
                  tunnel: [w215 w222 w229 w236 w243 w245] -> w207
                  tunnel: w210 -> [w216 w223 w230 w237 w243 w246]
                  tunnel: [State_Type_Definitions."Task 1" ("Enum") State_Type_Definitions."Task 2" ("Enum") State_Type_Definitions."Task 3" ("Enum") State_Type_Definitions."Task 4_A" ("Enum") State_Type_Definitions."Idle" ("Enum") State_Type_Definitions."Shutdown" ("Enum")] -> w209
                  frame "Start Task 1" {
                    n85 = for {
                      shift-right: [w220] -> w215
                      shift-left: w216 -> [w219]
                      tunnel: string[] ["RESET ENCODERS", "RESET YAW", "FORWARD", "READ ENCODERS"] -> [w218] mode=indexing
                      n86 = Enqueue Element(queue=w219, element=w218) -> (queue out=w220:refnum<queue>)  [unwired: 2 in, 2 out]
                    }
                  }
                  frame "Start Task 2" {
                    n87 = for {
                      shift-right: [w227] -> w222
                      shift-left: w223 -> [w226]
                      tunnel: string[] ["RESET ENCODERS", "RESET YAW", "ULTRASONIC READ", "ARDUINO MODE 0"] -> [w225] mode=indexing
                      n88 = Enqueue Element(queue=w226, element=w225) -> (queue out=w227:refnum<queue>)  [unwired: 2 in, 2 out]
                    }
                  }
                  frame "Start Task 3" {
                    n89 = for {
                      shift-right: [w234] -> w229
                      shift-left: w230 -> [w233]
                      tunnel: string[] ["RESET ENCODERS", "READ ENCODERS", "R-ACW"] -> [w232] mode=indexing
                      n90 = Enqueue Element(queue=w233, element=w232) -> (queue out=w234:refnum<queue>)  [unwired: 2 in, 2 out]
                    }
                  }
                  frame "Start Task 4" {
                    n91 = for {
                      shift-right: [w241] -> w236
                      shift-left: w237 -> [w240]
                      tunnel: string[] ["STOP", "RESET YAW", "RESET ENCODERS", "ARDUINO MODE 0", "ULTRASONIC READ", "FORWARD"] -> [w239] mode=indexing
                      n92 = Enqueue Element(queue=w240, element=w239) -> (queue out=w241:refnum<queue>)  [unwired: 2 in, 2 out]
                    }
                  }
                  frame "None", Default {
                  }
                  frame "Exit" {
                    n93 = for {
                      shift-right: [w250] -> w245
                      shift-left: w246 -> [w249]
                      tunnel: string[] ["STOP", "RESET ENCODERS", "RESET YAW", "EXIT"] -> [w248] mode=indexing
                      n94 = Enqueue Element(queue=w249, element=w248) -> (queue out=w250:refnum<queue>)  [unwired: 2 in, 2 out]
                    }
                  }
                }
              }
              frame 5 {
                n95 = for {
                  shift-right: [w258] -> w252
                  shift-left: w254 -> [w257]
                  tunnel: string[] ["INIT", "RESET ENCODERS", "RESET FLAGS", "EXIT"] -> [w256] mode=indexing
                  n96 = Enqueue Element(queue=w257, element=w256) -> (queue out=w258:refnum<queue>)  [unwired: 2 in, 2 out]
                }
              }
              frame 6 {
                n97 = Dequeue Element(queue=w271, timeout in ms (-1)=w270, error in (no error)=w269) -> (element=w268:T6)  [unwired: 3 out]
                n98 = Greater?(x=w262, y=250.0) -> (0:w260:bool)
                n99 = Or(x=w260, y=w263) -> (x .or. y?=w267:bool)
                n100 = case shown="\"Exit\"" w268 {
                  tunnel: w267 -> [w274 _]
                  tunnel: [w278 State_Type_Definitions."True Stop" ("Enum")] -> w266
                  tunnel: w265 -> [w275 w293]
                  tunnel: [w273 w292] -> w264
                  tunnel: [State_Type_Definitions."Idle" ("Enum") State_Type_Definitions."Shutdown" ("Enum")] -> w259
                  frame "None", Default {
                    n101 = case shown="True" w274 {
                      tunnel: w275 -> [w281 w287]
                      tunnel: [w280 w285] -> w273
                      frame False {
                        n102 = for {
                          shift-right: [w283] -> w280
                          shift-left: w281 -> [w284]
                          tunnel: string[] ["READ ENCODERS", "FORWARD"] ("element") -> [w282] mode=indexing
                          n103 = Enqueue Element(queue=w284, element=w282) -> (queue out=w283:refnum<queue>)  [unwired: 2 in, 2 out]
                        }
                      }
                      frame True {
                        n104 = for {
                          shift-right: [w289] -> w285
                          shift-left: w287 -> [w290]
                          tunnel: string[] ["RESET YAW", "RESET ENCODERS", "STOP", "ARDUINO MODE 0"] -> [w288] mode=indexing
                          n105 = Enqueue Element(queue=w290, element=w288) -> (queue out=w289:refnum<queue>)  [unwired: 2 in, 2 out]
                        }
                      }
                    }
                    n106 = Select(t=State_Type_Definitions."True Stop" ("Enum"), s=w274, f=State_Type_Definitions."Task 1" ("Enum")) -> (s? t:f=w278:u16)
                  }
                  frame "Exit" {
                    n107 = for {
                      shift-right: [w297] -> w292
                      shift-left: w293 -> [w298]
                      tunnel: string[] ["STOP", "RESET ENCODERS", "RESET YAW", ""] -> [w296] mode=indexing
                      n108 = Enqueue Element(queue=w298, element=w296) -> (queue out=w297:refnum<queue>)  [unwired: 2 in, 2 out]
                    }
                  }
                }
              }
              frame 7 {
                w307 = u16 20 ("y")
                # ">>Object detected>>"
                n109 = Dequeue Element(queue=w313, timeout in ms (-1)=w312, error in (no error)=w311) -> (element=w310:T6)  [unwired: 3 out]
                n110 = Less?(x=w309, y=w307) -> (x < y?=w306:bool)
                n111 = Less?(x=w308, y=w307) -> (x < y?=w305:bool)
                n112 = Or(x=w306, y=w305) -> (x .or. y?=w304:bool)
                "Object detected?" <- w304
                n113 = case shown="\"Exit\"" w310 {
                  tunnel: w304 -> [w317 _]
                  tunnel: [w319 State_Type_Definitions."True Stop" ("Enum")] -> w303
                  tunnel: w302 -> [w318 _]
                  tunnel: w301 -> [w316 w336]
                  tunnel: [w315 w337] -> w300
                  tunnel: [State_Type_Definitions."Idle" ("Enum") State_Type_Definitions."Shutdown" ("Enum")] -> w299
                  frame "None", Default {
                    n114 = case shown="True" w317 {
                      tunnel: w316 -> [w323 w330]
                      tunnel: [w324 w329] -> w315
                      frame False {
                        n115 = for {
                          tunnel: string[] ["ULTRASONIC READ", "STOP"] ("element") -> [w325] mode=indexing
                          shift-right: [w327] -> w324
                          shift-left: w323 -> [w326]
                          n116 = Enqueue Element(queue=w326, element=w325) -> (queue out=w327:refnum<queue>)  [unwired: 2 in, 2 out]
                        }
                      }
                      frame True {
                        n117 = for {
                          shift-right: [w332] -> w329
                          shift-left: w330 -> [w333]
                          tunnel: string[] ["REVERSE", "ULTRASONIC READ"] -> [w331] mode=indexing
                          n118 = Enqueue Element(queue=w333, element=w331) -> (queue out=w332:refnum<queue>)  [unwired: 2 in, 2 out]
                        }
                      }
                    }
                    n119 = Select(t=State_Type_Definitions."True Stop" ("Enum"), s=w318, f=State_Type_Definitions."Task 2" ("Enum")) -> (s? t:f=w319:u16)
                  }
                  frame "Exit" {
                    n120 = for {
                      shift-right: [w340] -> w337
                      shift-left: w336 -> [w341]
                      tunnel: string[] ["STOP", "RESET ENCODERS", "RESET YAW", "ARDUINO MODE 0"] -> [w339] mode=indexing
                      n121 = Enqueue Element(queue=w341, element=w339) -> (queue out=w340:refnum<queue>)  [unwired: 2 in, 2 out]
                    }
                  }
                }
              }
              frame 10 {
                n122 = Dequeue Element(queue=w354, timeout in ms (-1)=w353, error in (no error)=w352) -> (element=w343:T6)  [unwired: 3 out]
                n123 = Greater?(x=w351, y=150.0) -> (0:w348:bool)
                n124 = Or(x=w348, y=w349) -> (x .or. y?=w344:bool)
                n125 = case shown="\"Exit\"" w343 {
                  tunnel: w344 -> [w357 _]
                  tunnel: [w361 State_Type_Definitions."True Stop" ("Enum")] -> w345
                  tunnel: w347 -> [w358 w377]
                  tunnel: [w356 w376] -> w346
                  tunnel: [State_Type_Definitions."Idle" ("Enum") State_Type_Definitions."Shutdown" ("Enum")] -> w342
                  frame "None", Default {
                    n126 = case shown="False" w357 {
                      tunnel: w358 -> [w364 w370]
                      tunnel: [w363 w368] -> w356
                      frame False {
                        n127 = for {
                          shift-right: [w366] -> w363
                          shift-left: w364 -> [w367]
                          tunnel: string[] ["READ ENCODERS", "R-ACW"] ("element") -> [w365] mode=indexing
                          n128 = Enqueue Element(queue=w367, element=w365) -> (queue out=w366:refnum<queue>)  [unwired: 2 in, 2 out]
                        }
                      }
                      frame True {
                        n129 = for {
                          shift-right: [w372] -> w368
                          shift-left: w370 -> [w373]
                          tunnel: string[] ["RESET YAW", "RESET ENCODERS", "STOP", "ARDUINO MODE 0"] -> [w371] mode=indexing
                          n130 = Enqueue Element(queue=w373, element=w371) -> (queue out=w372:refnum<queue>)  [unwired: 2 in, 2 out]
                        }
                      }
                    }
                    n131 = Select(t=State_Type_Definitions."True Stop" ("Enum"), s=w357, f=State_Type_Definitions."Task 3" ("Enum")) -> (s? t:f=w361:T5)
                  }
                  frame "Exit" {
                    n132 = for {
                      shift-right: [w380] -> w376
                      shift-left: w377 -> [w381]
                      tunnel: string[] ["STOP", "RESET ENCODERS", "RESET YAW", ""] -> [w379] mode=indexing
                      n133 = Enqueue Element(queue=w381, element=w379) -> (queue out=w380:refnum<queue>)  [unwired: 2 in, 2 out]
                    }
                  }
                }
              }
              frame 11 {
                w386 = 50
                # ">> Outputs true if object detected >>"
                # ">> Manual override >>"
                n134 = Dequeue Element(queue=w395, timeout in ms (-1)=w394, error in (no error)=w393) -> (element=w392:T6)  [unwired: 3 out]
                n135 = Less?(x=w388, y=w386) -> (x < y?=w384:bool)
                n136 = Less?(x=w387, y=w386) -> (x < y?=w385:bool)
                n137 = And(x=w385, y=w384) -> (x .and. y?=w383:bool)
                n138 = case shown="\"None\", Default" w392 {
                  tunnel: [w405 State_Type_Definitions."True Stop" ("Enum")] -> w391
                  tunnel: [w403 w424] -> w390
                  tunnel: w396 -> [w402 _]
                  tunnel: w389 -> [w400 _]
                  tunnel: w383 -> [w398 _]
                  tunnel: [w397 State_Type_Definitions."Shutdown" ("Enum")] -> w382
                  frame "None", Default {
                    # ">> WIill proceed to part ii if not manual override >>"
                    # ">>If ENABLE or Trigger is set to true>>"
                    n139 = Or(x=w398, y=w400) -> (x .or. y?=w399:bool)
                    n140 = case shown="True" w399 {
                      tunnel: [w412 w417] -> w403
                      tunnel: w402 -> [w410 w416]
                      frame False {
                        n141 = for {
                          shift-right: [w414] -> w412
                          shift-left: w410 -> [w415]
                          tunnel: string[] ["FORWARD", "ULTRASONIC READ", ""] ("element") -> [w413] mode=indexing
                          n142 = Enqueue Element(queue=w415, element=w413) -> (queue out=w414:refnum<queue>)  [unwired: 2 in, 2 out]
                        }
                      }
                      frame True {
                        n143 = for {
                          shift-right: [w420] -> w417
                          shift-left: w416 -> [w421]
                          tunnel: string[] ["STOP", "RESET ENCODERS", "RESET YAW", "ARDUINO MODE 0"] -> [w419] mode=indexing
                          n144 = Enqueue Element(queue=w421, element=w419) -> (queue out=w420:refnum<queue>)  [unwired: 2 in, 2 out]
                        }
                      }
                    }
                    n145 = case shown="False" w400 {
                      tunnel: [State_Type_Definitions."True Stop" ("Enum") State_Type_Definitions."True Stop" ("Enum")] -> w401
                      tunnel: [State_Type_Definitions."Task 4_B" ("Enum") State_Type_Definitions."Idle" ("Enum")] -> w397
                      frame False {
                      }
                      frame True {
                      }
                    }
                    n146 = Select(t=w401, s=w399, f=State_Type_Definitions."Task 4_A" ("Enum")) -> (s? t:f=w405:T5)
                  }
                  frame "Exit" {
                    n147 = for {
                      shift-right: [w427] -> w424
                      shift-left: _ -> [w428]
                      tunnel: string[] ["STOP", "RESET ENCODERS", "RESET YAW", ""] -> [w426] mode=indexing
                      n148 = Enqueue Element(queue=w428, element=w426) -> (queue out=w427:refnum<queue>)  [unwired: 2 in, 2 out]
                    }
                  }
                }
              }
              frame 12 {
                w439 = 20
                # ">> Outputs true if 150 mm has been moved >>"
                # ">> Outputs true if sensor not obstructed>>"
                # ">> Manual override >>"
                n149 = Dequeue Element(queue=w444, timeout in ms (-1)=w443, error in (no error)=w442) -> (element=w441:T6)  [unwired: 3 out]
                n150 = Greater?(x=w436, y=w439) -> (0:w437:bool)
                n151 = Greater?(x=w435, y=w439) -> (0:w438:bool)
                n152 = Greater Or Equal?(x=w431, y=25.0) -> (x >= y?=w433:bool)
                n153 = And(x=w438, y=w437) -> (x .and. y?=w432:bool)
                n154 = And(x=w433, y=w432) -> (x .and. y?=w429:bool)
                n155 = case shown="\"None\", Default" w441 {
                  tunnel: [w456 State_Type_Definitions."True Stop" ("Enum")] -> w446
                  tunnel: [w454 w475] -> w447
                  tunnel: w440 -> [w453 _]
                  tunnel: w445 -> [w451 _]
                  tunnel: w429 -> [w449 _]
                  tunnel: [w448 State_Type_Definitions."Shutdown" ("Enum")] -> w430
                  frame "None", Default {
                    # ">> WIill proceed to part ii if not manual override >>"
                    # ">>If ENABLE or Trigger is set to true>>"
                    n156 = Or(x=w449, y=w451) -> (x .or. y?=w450:bool)
                    n157 = case shown="False" w450 {
                      tunnel: [w463 w468] -> w454
                      tunnel: w453 -> [w461 w467]
                      frame False {
                        n158 = for {
                          shift-right: [w465] -> w463
                          shift-left: w461 -> [w466]
                          tunnel: string[] ["RIGHT", "ULTRASONIC READ", "READ ENCODERS"] ("element") -> [w464] mode=indexing
                          n159 = Enqueue Element(queue=w466, element=w464) -> (queue out=w465:refnum<queue>)  [unwired: 2 in, 2 out]
                        }
                      }
                      frame True {
                        n160 = for {
                          shift-right: [w471] -> w468
                          shift-left: w467 -> [w472]
                          tunnel: string[] ["STOP", "RESET ENCODERS", "RESET YAW", "ARDUINO MODE 0"] -> [w470] mode=indexing
                          n161 = Enqueue Element(queue=w472, element=w470) -> (queue out=w471:refnum<queue>)  [unwired: 2 in, 2 out]
                        }
                      }
                    }
                    n162 = case shown="False" w451 {
                      tunnel: [State_Type_Definitions."True Stop" ("Enum") State_Type_Definitions."True Stop" ("Enum")] -> w452
                      tunnel: [State_Type_Definitions."Idle" ("Enum") State_Type_Definitions."Idle" ("Enum")] -> w448
                      frame False {
                      }
                      frame True {
                      }
                    }
                    n163 = Select(t=w452, s=w450, f=State_Type_Definitions."Task 4_B" ("Enum")) -> (s? t:f=w456:T5)
                  }
                  frame "Exit" {
                    n164 = for {
                      shift-right: [w478] -> w475
                      shift-left: _ -> [w479]
                      tunnel: string[] ["STOP", "RESET ENCODERS", "RESET YAW", ""] -> [w477] mode=indexing
                      n165 = Enqueue Element(queue=w479, element=w477) -> (queue out=w478:refnum<queue>)  [unwired: 2 in, 2 out]
                    }
                  }
                }
              }
              frame 13 {
                w492 = 30
                # ">> Outputs true if object detected >>"
                # ">> Manual override >>"
                n166 = Dequeue Element(queue=w482) -> (element=w493:T6)  [unwired: 2 in, 3 out]
                n167 = Less?(x=w487, y=w492) -> (x < y?=w490:bool)
                n168 = Less?(x=w488, y=w492) -> (x < y?=w491:bool)
                n169 = And(x=w491, y=w490) -> (x .and. y?=w489:bool)
                n170 = case shown="\"None\", Default" w493 {
                  tunnel: [w502 State_Type_Definitions."True Stop" ("Enum")] -> w483
                  tunnel: [w500 w523] -> w484
                  tunnel: w489 -> [w494 _]
                  tunnel: [w497 State_Type_Definitions."Shutdown" ("Enum")] -> w485
                  tunnel: w486 -> [w496 _]
                  tunnel: w481 -> [w495 w519]
                  tunnel: [w494 FALSE] -> w480
                  frame "None", Default {
                    # ">> WIill proceed to part ii if not manual override >>"
                    # ">>If ENABLE or Trigger is set to true>>"
                    n171 = Or(x=w494, y=w496) -> (x .or. y?=w498:bool)
                    n172 = case shown="True" w498 {
                      tunnel: [w509 w514] -> w500
                      tunnel: w495 -> [w507 w513]
                      frame False {
                        n173 = for {
                          shift-right: [w511] -> w509
                          shift-left: w507 -> [w512]
                          tunnel: string[] ["FORWARD", "ULTRASONIC READ", ""] ("element") -> [w510] mode=indexing
                          n174 = Enqueue Element(queue=w512, element=w510) -> (queue out=w511:refnum<queue>)  [unwired: 2 in, 2 out]
                        }
                      }
                      frame True {
                        n175 = for {
                          shift-right: [w517] -> w514
                          shift-left: w513 -> [w518]
                          tunnel: string[] ["STOP", "RESET ENCODERS", "RESET YAW", "ARDUINO MODE 0"] -> [w516] mode=indexing
                          n176 = Enqueue Element(queue=w518, element=w516) -> (queue out=w517:refnum<queue>)  [unwired: 2 in, 2 out]
                        }
                      }
                    }
                    n177 = case shown="True" w494 {
                      tunnel: [State_Type_Definitions."True Stop" ("Enum") State_Type_Definitions."True Stop" ("Enum")] -> w499
                      tunnel: [State_Type_Definitions."Idle" ("Enum") State_Type_Definitions."Idle" ("Enum")] -> w497
                      frame False {
                      }
                      frame True {
                      }
                    }
                    n178 = Select(t=w499, s=w498, f=State_Type_Definitions."Task 4_C" ("Enum")) -> (s? t:f=w502:T5)
                  }
                  frame "Exit" {
                    n179 = for {
                      shift-right: [w526] -> w523
                      shift-left: w519 -> [w527]
                      tunnel: string[] ["STOP", "RESET ENCODERS", "RESET YAW", ""] -> [w525] mode=indexing
                      n180 = Enqueue Element(queue=w527, element=w525) -> (queue out=w526:refnum<queue>)  [unwired: 2 in, 2 out]
                    }
                  }
                }
                "Object detected?" <- w480
              }
            }
          }
        }
      }
      n181 = call <vilib>:"NavX Close.vi"("NavX Info In"=w17) -> ()  [unwired: 10 in, 1 out]
      n182 = call <vilib>:"DIO Close.vi"("error in (no error)"=w2, "DIO Info In"=w5) -> ()  [unwired: 9 in, 1 out]
      n183 = call <vilib>:"DIO Close.vi"("error in (no error)"=w12, "DIO Info In"=w14) -> ()  [unwired: 9 in, 1 out]
      n184 = call <vilib>:"DIO Close.vi"("error in (no error)"=w7, "DIO Info In"=w9) -> ()  [unwired: 9 in, 1 out]
      n185 = Merge Errors "Merge Errors"(w44, w43) -> (w26:errorcluster)
      n186 = Merge Errors(w30, w26) -> (w24:errorcluster)
      n187 = Destroy User Event(user event=w47, error in=w24) -> ()  [unwired: 1 out]
      n188 = Destroy User Event(user event=w48, error in=w24) -> ()  [unwired: 1 out]
      n189 = Unregister For Events(event registration refnum=w39, error in=w24) -> ()  [unwired: 1 out]
      n190 = Release Queue(queue=w20, error in (no error)=w24) -> (error out=→"error out":errorcluster)  [unwired: 1 in, 2 out]
      n191 = Release Queue(queue=w38, error in (no error)=w24) -> ()  [unwired: 1 in, 3 out]
    }
    frame #2 {
      n192 = Wait (ms)(milliseconds to wait=u32 100) -> ()  [unwired: 1 out]
    }
  }
